vi "LoadBMP.vi"(8 "No Error":errorcluster, 11 "File":path) -> (0 "error out":errorcluster, 3 "surface [SDL_Surface *]":i64 format="%.0x")   [LabVIEW 2024, in "SDL3.lvlib" / "Surface.lvlib"]
doc: "<B>Summary</B>\nLoad a BMP image from a file.\n\n<B>Remarks</B>\nThe new surface should be freed with SDL_DestroySurface(). Not doing so will result in a memory leak."
uses:
  Surface.lvlib
  Lib/Win32/SDL3.dll
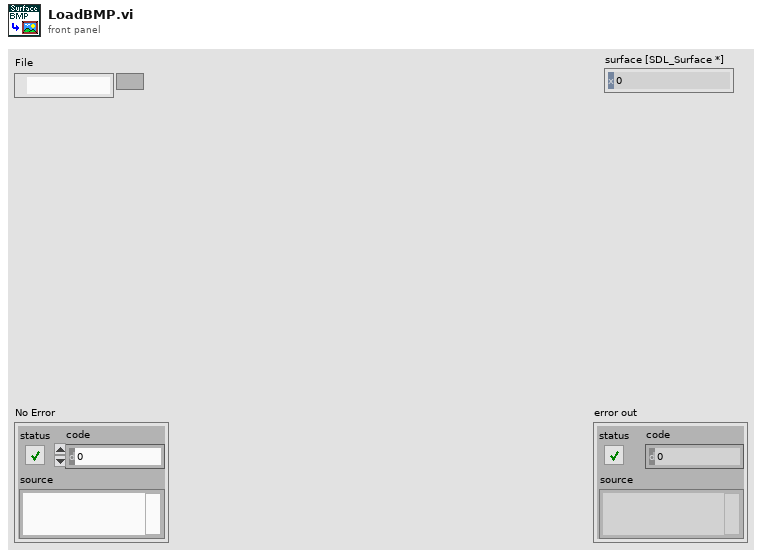
[diagram p1: front panel]
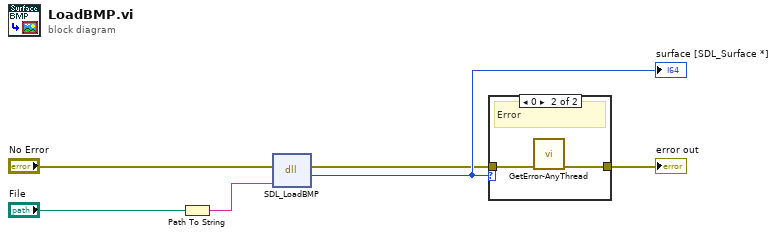
[diagram p0: block diagram]
diagram:
  n1 = Path To String(path="File") -> (string=w1:string)
  n2 = dll-call lib="C:/Users/Thomas/Documents/Projects/LV-SDL3/Lib/Win32/SDL3.dll" fn="SDL_LoadBMP"(error in="No Error", "file"=w1) -> (error out=w2:errorcluster, "return type"=w4:i64)  [unwired: 3 in, 1 out]
  "surface [SDL_Surface *]" <- w4
  n3 = case shown="0" w4 {
    tunnel: w2 -> [w7 w9]
    tunnel: [w7 w8] -> w5
    frame Default {
      # "Ok"
    }
    frame 0 {
      # "Error"
      n4 = call "GetError-AnyThread.vi"("No Error"=w9) -> ("Error Out"=w8:errorcluster)  [unwired: 10 in]
    }
  }
  "error out" <- w5
